vi "Item_OnPopupMenu.vi"(11 "Item Ref":T1) -> ()   [LabVIEW 2020, in "Negentropic IDE.lvlib"]
uses:
  Negentropic IDE.lvlib
  <resource>/Framework/Providers/API/ItemRef.ctl
  <resource>/Framework/Providers/API/mxLvMenuItem.ctl
  <vilib>/Utility/config.llb/Read Key (String).vi
  <vilib>/Utility/config.llb/NI_LVConfig.lvlib
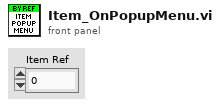
[diagram p1: front panel]
types:
  T1 = typedef "ItemRef.ctl" = u64
  T2 = typedef "mxLvMenuItem.ctl" = cluster{"Menu Name":string, "Description":string, "Icon File Name":path, "Menu Tag":string, "Enabled":bool, "Checked":bool, "Separator":bool, "Batchable":bool, "Weight":i32, "Batch Mode (Ignored if Not Batchable)":enum32{"Show If All Items Support Command", "Show If Any Items Support Command"}, "Menu Location":enum32{"<None>", "Project", "Project / Build Specifications", "Tools", "Tools / Source Control", "Tools / Real-Time Module", "Help"}, "Exclude From Getting Started Window Menu":bool}
  T3 = typedef "NI_LVConfig.lvlib/Config Data RefNum.ctl" = refnum<k1>
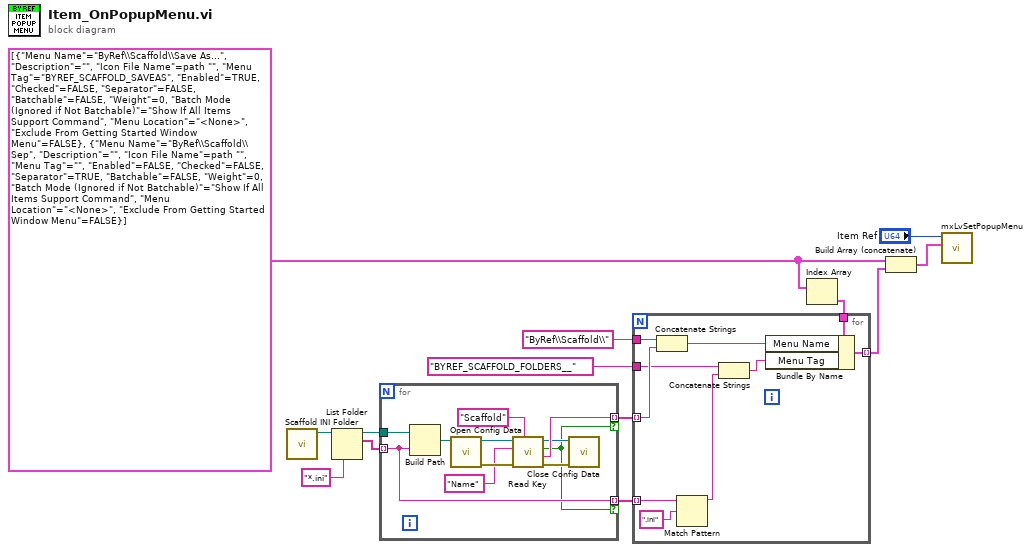
[diagram p0: block diagram]
diagram:
  w6 = T2[] [{"Menu Name"="ByRef\\Scaffold\\Save As...", "Description"="", "Icon File Name"=path "", "Menu Tag"="BYREF_SCAFFOLD_SAVEAS", "Enabled"=TRUE, "Checked"=FALSE, "Separator"=FALSE, "Batchable"=FALSE, "Weight"=0, "Batch Mode (Ignored if Not Batchable)"=enum."Show If All Items Support Command", "Menu Location"=enum."<None>", "Exclude From Getting Started Window Menu"=FALSE}, {"Menu Name"="ByRef\\Scaffold\\Sep", "Description"="", "Icon File Name"=path "", "Menu Tag"="", "Enabled"=FALSE, "Checked"=FALSE, "Separator"=TRUE, "Batchable"=FALSE, "Weight"=0, "Batch Mode (Ignored if Not Batchable)"=enum."Show If All Items Support Command", "Menu Location"=enum."<None>", "Exclude From Getting Started Window Menu"=FALSE}] ("Popup Menu Items")
  n1 = call "Scaffold INI Folder.vi"() -> ("Scaffold INI Folder"=w12:path)  [unwired: 10 in, 1 out]
  n2 = List Folder(path=w12, pattern="*.ini") -> (path out=w10:path, filenames=w9:string[])  [unwired: 2 in, 2 out]
  n3 = for {
    tunnel: w10 -> [w24]
    tunnel: w9 -> [w15] mode=indexing
    tunnel: [w18] -> w8 mode=indexing if=w14
    tunnel: [w15] -> w4 mode=indexing if=w14
    n4 = Build Path(base path=w24, name or relative path=w15) -> (appended path=w23:path)
    n5 = call <vilib>:"Open Config Data.vi"("configuration file path"=w23) -> ("error out"=w21:errorcluster, "refnum"=w22:T3)  [unwired: 8 in, 1 out]
    n6 = call-poly <vilib>:"Read Key.vi"("section"="Scaffold", "error in (no error)"=w21, "key"="Name", "refnum"=w22) -> ("error out"=w16:errorcluster, "value"=w18:string, "found?"=w14:bool, "refnum out"=w17:T3)  [unwired: 4 in]
    n7 = call <vilib>:"Close Config Data.vi"("error in (no error)"=w16, "refnum"=w17) -> ()  [unwired: 8 in, 2 out]
  }
  n8 = Index Array(array=w6) -> (element=w5:T2)  [unwired: 1 in]
  n9 = for {
    tunnel: w8 -> [w33] mode=indexing
    tunnel: "ByRef\\Scaffold\\" -> [w34]
    tunnel: w5 -> [w32]
    tunnel: w4 -> [w30] mode=indexing
    tunnel: "BYREF_SCAFFOLD_FOLDERS__" -> [w28]
    tunnel: [w25] -> w1 mode=indexing
    n10 = Concatenate Strings(w34, w33) -> (w31:string)
    n11 = Match Pattern(string=w30, regular expression=".ini") -> (before substring=w27:string)  [unwired: 1 in, 3 out]
    n12 = Concatenate Strings(w28, w27) -> (w26:string)
    n13 = Bundle By Name(cluster=w32, "Menu Name"=w31, "Menu Tag"=w26) -> (w25:T2)
  }
  n14 = Build Array (concatenate)(w6, w1) -> (w2:T2[])
  n15 = call <resource>:"mxLvSetPopupMenu.vi"("Popup Menu Items"=w2, "Item"="Item Ref") -> ()  [unwired: 8 in, 2 out]
